vi "caxis_fine_fit.vi"(7 "Grain Number":i32, 8 "Error In":errorcluster, 9 "phic start":dbl, 10 "thetac start":dbl, 11 "Sample Results":T1) -> (0 "Error Out":errorcluster, 1 "Best R2":dbl, 2 "Theta min":dbl, 3 "Phi min":dbl)   [LabVIEW 2019]
uses:
  sample_results_cluster_typedef.ctl
  parameters_cluster_typedef.ctl
  writeable_section_parameters_cluster_typedef.ctl
  grain_results_cluster_typedef.ctl
  thetac_phic_enum_typedef.ctl
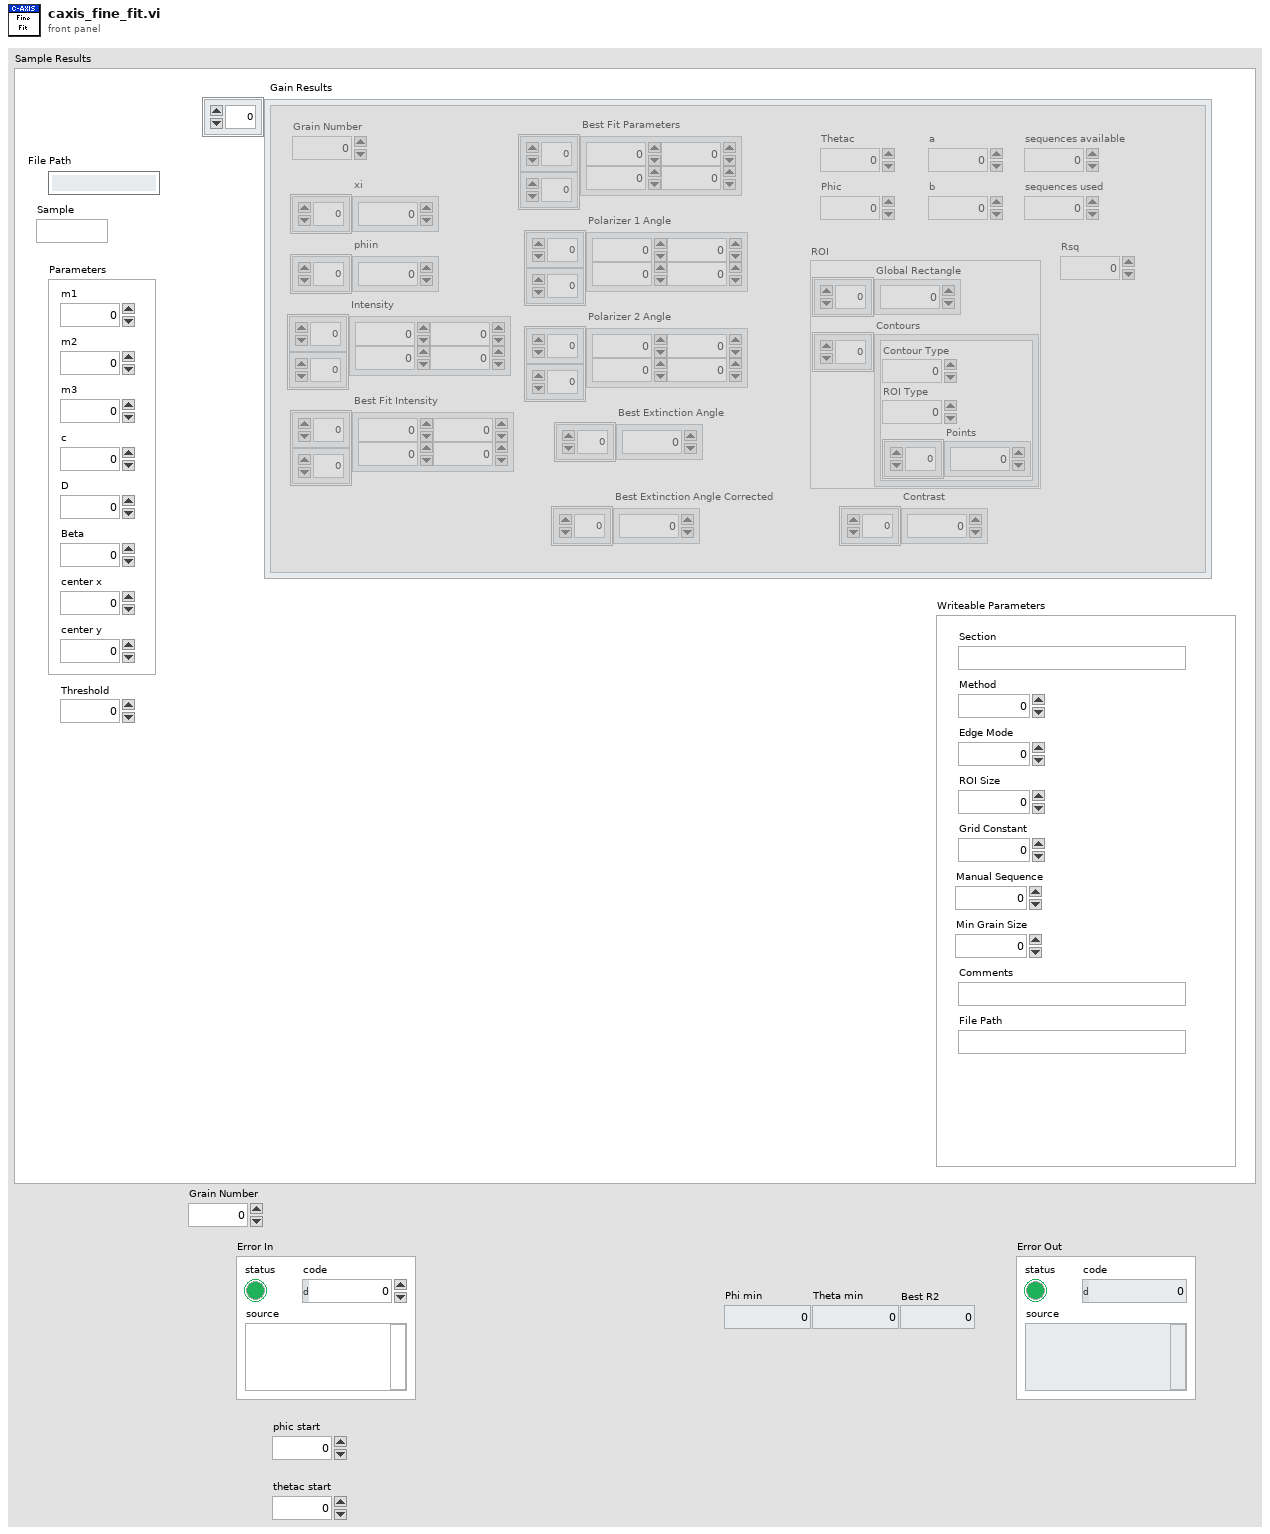
[diagram p1: front panel]
types:
  T1 = typedef "sample_results_cluster_typedef.ctl" = cluster{"File Path":string, "Sample":string, "Threshold":dbl, "Parameters":T2, "Writeable Parameters":T3, "Gain Results":T4[]}
  T2 = typedef "parameters_cluster_typedef.ctl" = cluster{"m1":dbl, "m2":dbl, "m3":dbl, "c":dbl, "D":dbl, "Beta":dbl, "center x":dbl, "center y":dbl}
  T3 = typedef "writeable_section_parameters_cluster_typedef.ctl" = cluster{"Section":string, "Method":i32, "Edge Mode":i32, "Grid Constant":i32, "Manual Sequence":i32, "ROI Size":i32, "Min Grain Size":dbl, "Comments":string, "File Path":string}
  T4 = typedef "grain_results_cluster_typedef.ctl" = cluster{"Grain Number":i32, "xi":dbl[], "phiin":dbl[], "Intensity":dbl[][], "Best Fit Intensity":dbl[][], "Best Fit Parameters":dbl[][], "Polarizer 1 Angle":dbl[][], "Polarizer 2 Angle":dbl[][], "Best Extinction Angle":dbl[], "Best Extinction Angle Corrected":dbl[], "Thetac":dbl, "Phic":dbl, "ROI":cluster{"Global Rectangle":i32[], "Contours":cluster{"Contour Type":u32, "ROI Type":u32, "Points":i32[]}[]}, "a":dbl, "b":dbl, "sequences available":dbl, "sequences used":dbl, "Contrast":dbl[], "Rsq":dbl}
  T5 = typedef "thetac_phic_enum_typedef.ctl" = enum16{"phic", "thetac"}
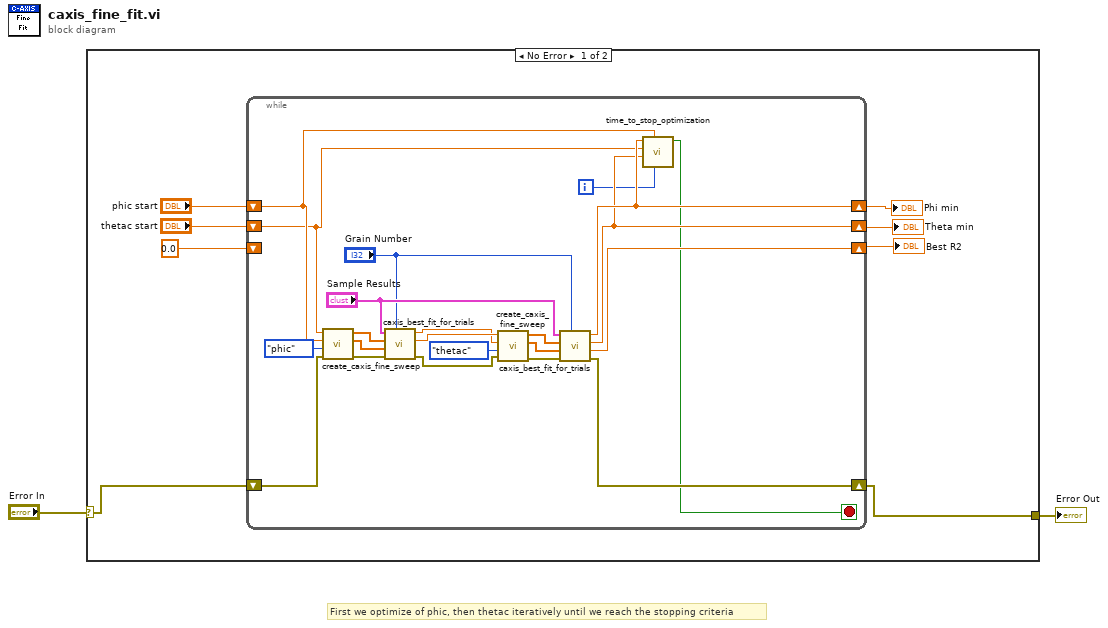
[diagram p0: block diagram]
diagram:
  # "First we optimize of phic, then thetac iteratively until we reach the stopping criteria"
  n1 = case shown="No Error" "Error In" {
    selector: "Error In" -> [w8 w33]
    tunnel: [w3 w33] -> w1
    frame No Error {
      n2 = while {
        shift-right: [w16] -> w5
        shift-left: "thetac start" -> [w14]
        shift-right: [w17] -> w6
        shift-left: "phic start" -> [w15]
        shift-right: [w18] -> w3
        shift-left: w8 -> [w32]
        shift-right: [w19] -> w4
        shift-left: 0.0 -> [_]
        i -> [w13]
        stop <- w12 stop-if-true
        n3 = call "create_caxis_fine_sweep.vi"("Error In"=w32, "Variable to Change"=thetac_phic_enum_typedef."phic", "phic center"=w15, "thetac center"=w14) -> ("Error Out"=w28:errorcluster, "phic"=w29:dbl[], "thetac"=w30:dbl[])  [unwired: 5 in]
        n4 = call "caxis_best_fit_for_trials.vi"("Grain Number"="Grain Number", "Error In"=w28, "phic"=w29, "thetac"=w30, "Sample Results"="Sample Results") -> ("Error Out"=w21:errorcluster, "Theta min"=w23:dbl, "Phi min"=w22:dbl)  [unwired: 3 in, 1 out]
        n5 = call "create_caxis_fine_sweep.vi"("Error In"=w21, "Variable to Change"=thetac_phic_enum_typedef."thetac", "phic center"=w22, "thetac center"=w23) -> ("Error Out"=w27:errorcluster, "phic"=w26:dbl[], "thetac"=w25:dbl[])  [unwired: 5 in]
        n6 = call "caxis_best_fit_for_trials.vi"("Grain Number"="Grain Number", "Error In"=w27, "phic"=w26, "thetac"=w25, "Sample Results"="Sample Results") -> ("Error Out"=w18:errorcluster, "Best R2"=w19:dbl, "Theta min"=w16:dbl, "Phi min"=w17:dbl)  [unwired: 3 in]
        n7 = call "time_to_stop_optimization.vi"("Iterations"=w13, "Previous Phic"=w15, "New Thetac"=w16, "Previous Thetac"=w14, "New Phic"=w17) -> ("Stop?"=w12:bool)  [unwired: 5 in, 1 out]
      }
      "Phi min" <- w6
      "Theta min" <- w5
      "Best R2" <- w4
    }
    frame Error {
    }
  }
  "Error Out" <- w1
